vi "Tosca-Locomotion Thread.vi"(0 "IPC":T1) -> (15 "error out":errorcluster)   [LabVIEW 2020]
uses:
  IPC VIs/Tosca-IPC.ctl
  Classes/Parameters/Parameters.lvclass
  Digital Input VIs/Tosca-DI Queue Data.ctl
  Digital Input VIs/Tosca-Input Event.ctl
  Digital Input VIs/Tosca-Input Criterion.ctl
  epl-vi-lib/Utility VIs/Type Defs/Logic State.ctl
  Typedefs/Tosca-Accumulator.ctl
  Typedefs/Tosca-State AODO.ctl
  Typedefs/Tosca-AO Runtime.ctl
  Typedefs/Tosca-DO Runtime.ctl
  epl-vi-lib/Signal Synthesis VIs/4th Generation/Classes/SignalManager/SignalManager.lvclass
  Typedefs/Tosca-Synapse Start Data.ctl
  IPC VIs/Tosca-Message.ctl
  IPC VIs/Tosca-Message Action.ctl
  Typedefs/Tosca-Thread Type.ctl
  Imaging VIs/Tosca-2P-Notifier Data.ctl
  Typedefs/Tosca-MATLAB Queue Data.ctl
  Visual Stim VIs/Tosca-Grating.ctl
  Visual Stim VIs/Tosca-Grating Type.ctl
  Typedefs/Tosca-File IO Notification.ctl
  Typedefs/Tosca-Locomotion Settings.ctl
  epl-vi-lib/TCP VIs/TCP Write.vi
  Sub VIs/Tosca-Globals.vi
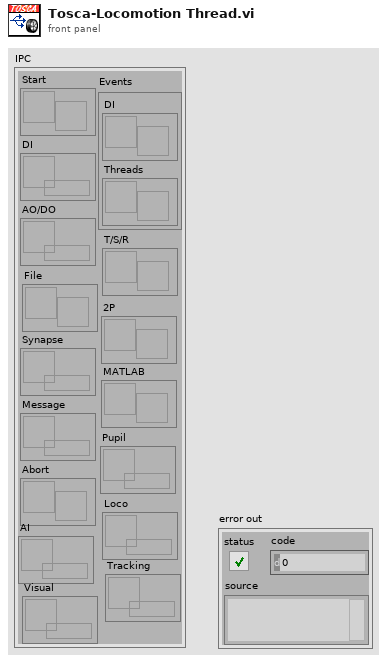
[diagram p1: front panel]
types:
  T1 = typedef "Tosca-IPC.ctl" = cluster{"Start":refnum<notifier>, "DI":refnum<queue>, "AO/DO":refnum<queue>, "Synapse":refnum<queue>, "Message":refnum<queue>, "Abort":refnum<notifier>, "Events":cluster{"DI":refnum<user-event>, "Threads ":refnum<user-event>}, "T/S/R":refnum<notifier>, "2P":refnum<notifier>, "MATLAB":refnum<notifier>, "Pupil":refnum<queue>, "Loco":refnum<queue>, "AI":refnum<queue>, "Tracking":refnum<queue>, "Visual":refnum<queue>, "File":refnum<notifier>}
  T2 = enum16{"big-endian, network order", "native, host order", "little-endian"}
  T3 = typedef "Tosca-Locomotion Settings.ctl" = cluster{"IP Address":string, "Port":i32, "Send markers":bool}
  T4 = typedef "Tosca-Thread Type.ctl" = enum16{"None", "AODO", "Masker", "ET", "Imaging", "Pupil", "AI", "DI", "Camera", "TTL out", "Loco", "Visual"}
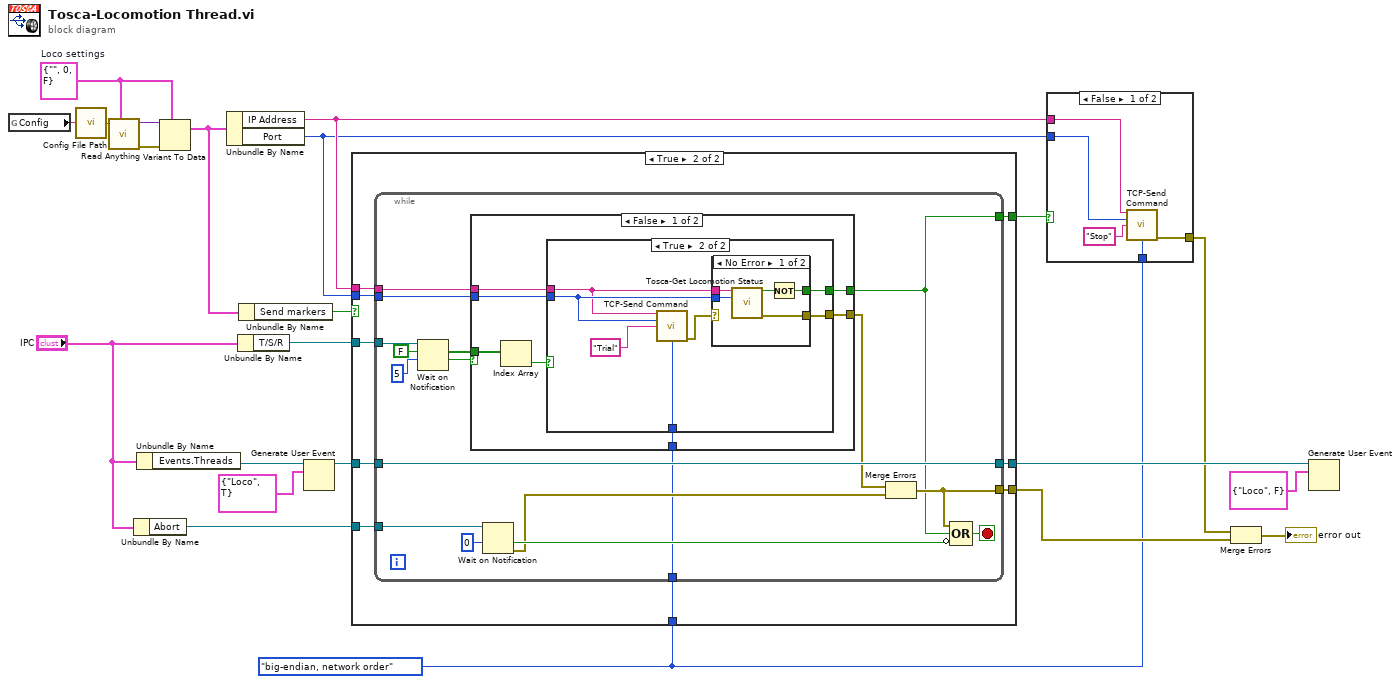
[diagram p0: block diagram]
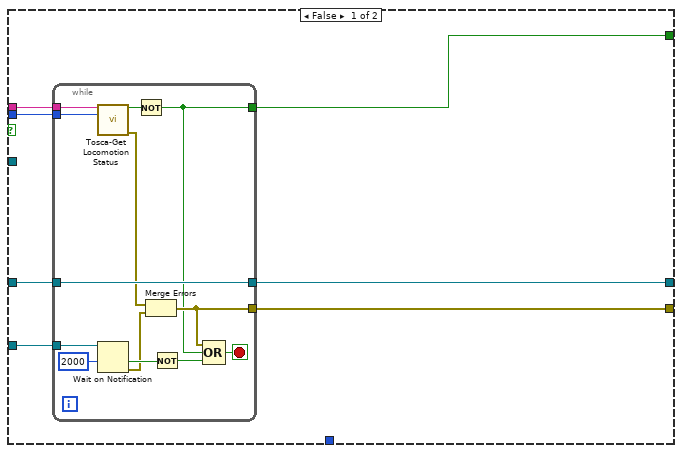
[diagram p2: hidden frame]
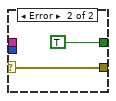
[diagram p4: hidden frame]
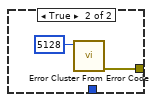
[diagram p6: hidden frame]
diagram:
  w1 = T2."big-endian, network order" ("byte order")
  w4 = T3 {"IP Address"="", "Port"=0, "Send markers"=FALSE}  # Loco settings
  n1 = global read "Tosca-Globals.vi" "Config"() -> (w7:string)
  n2 = call "Config File Path.vi"("AppName"=w7) -> ("Default config file name"=w14:path)
  n3 = call "Read Anything.vi"("Type of Anything"=w4, "Path (dialog)"=w14) -> ("Error Out"=w16:errorcluster, "Anything"=w15:variant)  [unwired: 7 in, 1 out]
  n4 = Unbundle By Name("IPC") -> ("Abort"=w17:refnum<notifier>)
  n5 = Unbundle By Name("IPC") -> ("Events.Threads"=w22:refnum<user-event>)
  n6 = Variant To Data(error in=w16, type=w4, Variant=w15) -> (data=w3:T3)  [unwired: 1 out]
  n7 = Unbundle By Name(w3) -> ("IP Address"=w9:string, "Port"=w8:i32)
  n8 = Unbundle By Name("IPC") -> ("T/S/R"=w5:refnum<notifier>)
  n9 = Unbundle By Name(w3) -> ("Send markers"=w2:bool)
  n10 = Generate User Event(user event=w22, event data cluster=cluster{"ID":T4, "Running":bool} {"ID"=enum."Loco", "Running"=TRUE} ("event data")) -> (user event out=w20:refnum<user-event>)  [unwired: 2 in, 1 out]
  n11 = case shown="True" w2 {
    tunnel: w20 -> [w29 w49]
    tunnel: [w28 w45] -> w19
    tunnel: w17 -> [w27 w48]
    tunnel: [w26 w46] -> w12
    tunnel: [w25 w44] -> w11
    tunnel: w9 -> [w24 w51]
    tunnel: w8 -> [w23 w50]
    tunnel: w5 -> [_ w47]
    tunnel: w1 -> [_ w43]
    frame False {
      n12 = while {
        tunnel: w29 -> [w42]
        tunnel: [w42] -> w28
        tunnel: w27 -> [w39]
        tunnel: w24 -> [w36]
        tunnel: w23 -> [w35]
        tunnel: [w30] -> w26
        tunnel: [w31] -> w25
        stop <- w37 stop-if-true
        n13 = call "Tosca-Get Locomotion Status.vi"("IP Address"=w36, "Port"=w35) -> ("Recording"=w34:bool, "error out"=w33:errorcluster)  [unwired: 12 in]
        n14 = Wait on Notification(notifier=w39, timeout in ms (-1)=2000) -> (timed out?=w41:bool, error out=w32:errorcluster)  [unwired: 2 in, 2 out]
        n15 = Not(x=w34) -> (.not. x?=w30:bool)
        n16 = Merge Errors(w33, w32) -> (w31:errorcluster)
        n17 = Not(x=w41) -> (.not. x?=w38:bool)
        n18 = Compound Arithmetic op=OR(w31, w30, w38) -> (w37:bool)
      }
    }
    frame True {
      n19 = while {
        tunnel: w49 -> [w68]
        tunnel: [w68] -> w45
        tunnel: w48 -> [w65]
        tunnel: w51 -> [w54]
        tunnel: w50 -> [w55]
        tunnel: [w61] -> w46
        tunnel: [w62] -> w44
        tunnel: w47 -> [w58]
        tunnel: w43 -> [w52]
        stop <- w64 stop-if-true
        n20 = Wait on Notification(notifier=w58, ignore previous (F)=FALSE, timeout in ms (-1)=5) -> (notification=w56:bool[], timed out?=w57:bool)  [unwired: 1 in, 2 out]
        n21 = case shown="False" w57 {
          tunnel: w56 -> [w74 _]
          tunnel: w54 -> [w73 _]
          tunnel: w55 -> [w72 _]
          tunnel: [w71 _] -> w53
          tunnel: [w70 _] -> w61
          tunnel: w52 -> [w69 _]
          frame False {
            n22 = Index Array(array=w74) -> (element=w75:bool)  [unwired: 1 in]
            n23 = case shown="True" w75 {
              tunnel: w73 -> [_ w80]
              tunnel: w72 -> [_ w81]
              tunnel: [_ w79] -> w71
              tunnel: [_ w78] -> w70
              tunnel: w69 -> [_ w76]
              frame False {
              }
              frame True {
                n24 = call "TCP-Send Command.vi"("PXI Address"=w80, "Port"=w81, "Command"="Trial" ("format string"), "byte order"=w76) -> ("error out"=w82:errorcluster)  [unwired: 11 in]
                n25 = case shown="No Error" w82 {
                  selector: w82 -> [_ w89]
                  tunnel: w81 -> [w85 _]
                  tunnel: w80 -> [w86 _]
                  tunnel: [w83 w89] -> w79
                  tunnel: [w87 TRUE ("Recording")] -> w78
                  frame No Error {
                    n26 = call "Tosca-Get Locomotion Status.vi"("IP Address"=w86, "Port"=w85) -> ("Recording"=w84:bool, "error out"=w83:errorcluster)  [unwired: 12 in]
                    n27 = Not(x=w84) -> (.not. x?=w87:bool)
                  }
                  frame Error {
                  }
                }
              }
            }
          }
          frame True {
          }
        }
        n28 = Wait on Notification(notifier=w65, timeout in ms (-1)=0) -> (timed out?=w67:bool, error out=w63:errorcluster)  [unwired: 2 in, 2 out]
        n29 = Merge Errors(w53, w63) -> (w62:errorcluster)
        n30 = Compound Arithmetic op=OR(w62, w61, invert w67) -> (w64:bool)
      }
    }
  }
  n31 = case shown="False" w12 {
    tunnel: [w91 w95] -> w10
    tunnel: w9 -> [w93 _]
    tunnel: w8 -> [w92 _]
    tunnel: w1 -> [w90 _]
    frame False {
      n32 = call "TCP-Send Command.vi"("PXI Address"=w93, "Port"=w92, "Command"="Stop", "byte order"=w90) -> ("error out"=w91:errorcluster)  [unwired: 11 in]
    }
    frame True {
      n33 = call <vilib>:"Error Cluster From Error Code.vi"("error code (0)"=5128) -> ("error out"=w95:errorcluster)  [unwired: 8 in]
    }
  }
  n34 = Merge Errors(w10, w11) -> (→"error out":errorcluster)
  n35 = Generate User Event(user event=w19, event data cluster=cluster{"ID":T4, "Running":bool} {"ID"=enum."Loco", "Running"=FALSE} ("event data")) -> ()  [unwired: 2 in, 2 out]
